vi "zadanie_2.vi"() -> ()   [LabVIEW 2020]
panel:
  out "Numeric 4":dbl
  out "Numeric 3":dbl
  out "Numeric 2":dbl
  out "Numeric":dbl
  out "System dziesietny":dbl
  in  "1":bool
  in  "2":bool
  in  "4":bool
  in  "8":bool
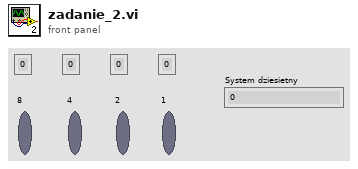
[diagram p1: front panel]
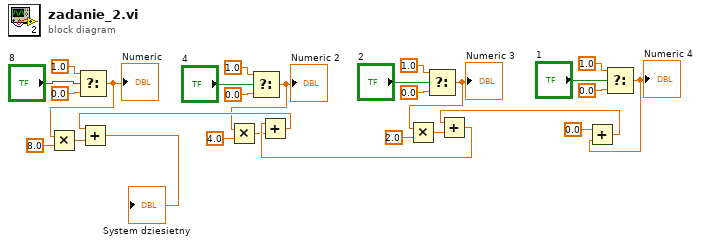
[diagram p0: block diagram]
diagram:
  n1 = Select(t=1.0, s="8", f=0.0) -> (s? t:f=w2:dbl)
  "Numeric" <- w2
  n2 = Multiply(x=w2, y=8.0) -> (x*y=w6:dbl)
  n3 = Select(t=1.0, s="4", f=0.0) -> (s? t:f=w3:dbl)
  "Numeric 2" <- w3
  n4 = Multiply(x=w3, y=4.0) -> (x*y=w7:dbl)
  n5 = Select(t=1.0, s="2", f=0.0) -> (s? t:f=w9:dbl)
  "Numeric 3" <- w9
  n6 = Multiply(x=w9, y=2.0) -> (x*y=w10:dbl)
  n7 = Select(t=1.0, s="1", f=0.0) -> (s? t:f=w8:dbl)
  "Numeric 4" <- w8
  n8 = Add(x=0.0, y=w8) -> (x+y=w1:dbl)
  n9 = Add(x=w1, y=w10) -> (x+y=w15:dbl)
  n10 = Add(x=w15, y=w7) -> (x+y=w14:dbl)
  n11 = Add(x=w14, y=w6) -> (x+y=→"System dziesietny":dbl)
